vi "HFRR ADV v10.vi"() -> ()   [LabVIEW 2025] (continued)
            n1538 = Add(x=w2006, y=w2020) -> (x+y=w2022:dbl)
            n1539 = call-poly <vilib>:"Mean.vi"("X"=w2043) -> ("mean"=w2044:dbl)  [unwired: 1 out]
            n1540 = Add(x=w1991, y=w1992) -> (x+y=w1990:dbl)
            n1541 = Subtract(x=1.0 ("y"), y=w2032) -> (x-y=w2030:dbl)
            n1542 = local write "TEMP"(w1982) -> ()
            n1543 = Multiply(x=w2030, y=w2029) -> (x*y=w2028:dbl)
            n1544 = Multiply(x=w2022, y=w2032) -> (x*y=w2033:dbl)
            n1545 = Not A Number/Path/Refnum?(number/path/refnum=w1990) -> (NaN/Path/Refnum?=w2000:bool)
            n1546 = Subtract(x=w2043, y=w2044) -> (x-y=w2015:dbl[])
            n1547 = local read "FRICVALZ"() -> (w2053:dbl)
            n1548 = case shown="True" "Camera Button" {
              tunnel: w2010 -> [_ w2072]
              tunnel: "Standard Temp. ( °c )" -> [_ w2071]
              frame False {
              }
              frame True {
                n1549 = Build Array(w2071, w2072) -> (w2070:dbl[])
                n1550 = local write "Camera Button"(FALSE ("Boolean 4")) -> ()
                n1551 = local read "Captured Values"() -> (w2069:dbl[][])
                n1552 = Build Array (concatenate)(w2069, w2070) -> (w2067:dbl[][])
                n1553 = local write "Captured Values"(w2067) -> ()
              }
            }
            n1554 = Compound Arithmetic op=OR("FRICVALZ 4", "FRICVALZ 3", "FRICVALZ 2") -> (w1984:bool)
            n1555 = Add(x=w2033, y=w2028) -> (x+y=w2026:dbl)
            n1556 = Absolute Value(x=w2015) -> (abs(x)=w2048:dbl[])
            n1557 = call-poly <vilib>:"RMS.vi"("X"=w2015) -> ("rms value"=w2014:dbl)  [unwired: 1 out]
            n1558 = Select(t=0.0, s=w2000, f=w1990) -> (s? t:f=w1997:dbl)
            n1559 = call-poly <vilib>:"Mean.vi"("X"=w2048) -> ()  [unwired: 2 out]
            n1560 = local read "FF 2"() -> (w2055:dbl)
            n1561 = case shown="True" w1984 {
              tunnel: w2014 -> [_ w2077]
              frame False {
              }
              frame True {
                w2076 = FALSE ("FRICVALZ")
                n1562 = local write "FRICVALZ 3"(w2076) -> ()
                n1563 = local write "FRICVALZ 2"(w2076) -> ()
                n1564 = local write "FRICVALZ 4"(w2076) -> ()
                "FRICVALZ" <- w2077
              }
            }
            n1565 = Subtract(x=w2014, y=w2053) -> (x-y=w2047:dbl)
            n1566 = Not A Number/Path/Refnum?(number/path/refnum=w2026) -> (NaN/Path/Refnum?=w2027:bool)
            n1567 = In Range and Coerce(upper limit=100.0, x=w1997, lower limit=0.0) -> ()  [unwired: 2 out]
            n1568 = Select(t=0.0, s=w2027, f=w2026) -> (s? t:f=w1987:dbl)
            "AIR TEMP" <- w1987
            n1569 = Multiply(x=w2047, y=0.1 ("FF fil1")) -> (x*y=w2059:dbl)
            n1570 = Multiply(x=0.9 ("FF fil2"), y=w2055) -> (x*y=w2058:dbl)
            n1571 = disable-structure shown="Disabled" {
              frame Disabled {
                n1572 = local read "NORMAL LOAD"() -> ()  [unwired: 1 out]
              }
              frame Enabled {
              }
            }
            n1573 = call "Elapsed Time11"("Time Target (s)"=1.0) -> ("Time has Elapsed"=w1989:bool)  [unwired: 11 in, 7 out]
            n1574 = Add(x=w2059, y=w2058) -> (x+y=w1977:dbl)
            "FF 2" <- w1977
            "FF 4" <- w1977
            n1575 = case shown="True" w1989 {
              tunnel: w1987 -> [_ w2061]
              frame False {
              }
              frame True {
                "AirT" <- w2061
              }
            }
            n1576 = local read "TEMP"() -> (w2052:dbl)
            n1577 = local write "FF 3"(w1977) -> ()
            n1578 = Not A Number/Path/Refnum?(number/path/refnum=w1977) -> (NaN/Path/Refnum?=w2050:bool)
            n1579 = Divide(x=w1977, y=1.96) -> (x/y=w2017:dbl)
            n1580 = Not A Number/Path/Refnum?(number/path/refnum=w2052) -> (NaN/Path/Refnum?=w2051:bool)
            n1581 = Compound Arithmetic op=OR(w2051, w2050) -> (w2049:bool)
            n1582 = Not A Number/Path/Refnum?(number/path/refnum=w2017) -> (NaN/Path/Refnum?=w2018:bool)
            n1583 = case shown="True" w2049 {
              frame False {
              }
              frame True {
                n1584 = local write "TEMP"(0.0 ("TEMP")) -> ()
                n1585 = local write "FF 2"(0.0 ("FF 2")) -> ()
                n1586 = local write "reinit"(TRUE ("reinit")) -> ()
              }
            }
            n1587 = Select(t=0.0, s=w2018, f=w2017) -> (s? t:f=w1978:dbl)
            "COF 2" <- w1978
            n1588 = local write "COF 3"(w1978) -> ()
          }
          frame #4 {
            n1589 = flat-sequence {
              frame #0 {
                n1590 = Wait (ms)(milliseconds to wait=u32 100) -> ()  [unwired: 1 out]
              }
              frame #1 {
                n1591 = local write "Lift"(FALSE ("Lift")) -> ()
              }
            }
            n1592 = case shown="True" "Calculate Button" {
              frame False {
              }
              frame True {
                n1593 = local write "Calculate Button"(FALSE ("Boolean 6")) -> ()
                n1594 = local read "Captured Values"() -> (w2088:dbl[][])
                n1595 = Index Array(array=w2088, index (col) #1=0 ("disabled index (col)"), index (col) #2=1 ("index (col)")) -> (element #1=w2086:dbl[], element #2=w2084:dbl[])  [unwired: 2 in]
                n1596 = call <vilib>:"Linear Fit.vi"("Y"=w2086, "X"=w2084) -> ("Best Linear Fit"=→"Best Fit":dbl[], "slope"=w2080:dbl, "intercept"=w2079:dbl)  [unwired: 9 in, 2 out]
                "Slope" <- w2080
                "Intercept" <- w2079
                n1597 = local read "Calibrating"() -> (w2081:string)
                n1598 = case shown="\"1\"" w2081 {
                  tunnel: w2080 -> [w2090 w2092]
                  tunnel: w2079 -> [w2089 w2091]
                  frame "0", Default {
                    n1599 = local write "TEMPERATURE :"(w2090) -> ()
                    n1600 = local write "TEMP INTERCEPT:"(w2089) -> ()
                  }
                  frame "1" {
                    n1601 = local write "AIR TEMPERATURE :"(w2092) -> ()
                    n1602 = local write "AIR TEMP INTERCEPT:"(w2091) -> ()
                  }
                }
              }
            }
          }
        }
      }
    }
    n1603 = Wait (ms)(milliseconds to wait=u32 50) -> ()  [unwired: 1 out]
    n1604 = local read "Quit"() -> (w1882:bool)
    "Rate" <- 2500.0 ("No of Samples")
    "Humid Last buf" <- dbl[] [0.0, 0.0, 0.0, 0.0] ("Humid Last buf")
  }
  n1605 = while {
    tunnel: w60 -> [_]
    tunnel: [w2122] -> _
    tunnel: [w2097] -> w57
    i -> [w2122]
    stop <- w2097 stop-if-true
    # "C:\\LAB-IQ-NXT\\Scar View.exe"
    n1606 = local read "OK Button 16"() -> (w2111:bool)
    n1607 = local read "Re-Initialise"() -> (w2107:bool)
    n1608 = local read "Main Tab"() -> (w2103:T2)
    n1609 = local read "service 3"() -> (w2104:bool)
    n1610 = local read "OPEN 6"() -> (w2106:bool)
    n1611 = local read "EDIT 2"() -> (w2109:bool)
    n1612 = flat-sequence {
      frame #0 {
        n1613 = local read "SAVE 2"() -> (w2725:bool)
        n1614 = stacked-sequence {
          frame #0 {
            n1615 = local read "EDIT"() -> (w2779:bool)
            n1616 = case shown="True" w2779 {
              tunnel: [u8 2 ("Disabled") u8 0 ("Disabled")] -> _
              frame False {
                w2781 = FALSE
                n1617 = local write "Password"("") -> ()
                n1618 = property on="SrvM CP" class="Bool (strict)"("Visible"=w2781) -> ()  [unwired: 2 in, 2 out]
                n1619 = property on="message" class="Str"("Visible"=w2781) -> ()  [unwired: 2 in, 2 out]
                n1620 = local write "x = y?"(w2781) -> ()
                n1621 = property on="Password" class="Str"("Visible"=w2781) -> ()  [unwired: 2 in, 2 out]
                n1622 = property on="ENTER THE NEW PASSWORD" class="Str"("Visible"=w2781) -> ()  [unwired: 2 in, 2 out]
                n1623 = property on="ENTER CURRENT PASSWORD" class="Str"("Visible"=w2781) -> ()  [unwired: 2 in, 2 out]
                n1624 = local write "SrvM CP"(w2781) -> ()
              }
              frame True {
                w2784 = TRUE
                n1625 = property on="SrvM CP" class="Bool (strict)"("Visible"=w2784) -> ()  [unwired: 2 in, 2 out]
                n1626 = property on="Password" class="Str"("Visible"=w2784) -> ()  [unwired: 2 in, 2 out]
              }
            }
            "dipl pwd" <- "@143$\n" ("dipl pwd")
          }
          frame #1 {
            # "Gain password"
            n1627 = String To Byte Array(string="ENTER CURRENT PASSWORD") -> (unsigned byte array=w2789:u8[])
            n1628 = Search 1D Array(1D array=w2789, element=u8 10) -> (index of element=w2792:i32)  [unwired: 1 in]
            n1629 = Index Array(array=w2789, index=w2792) -> (element=w2788:u8)
            n1630 = Equal?(x=w2788, y=10) -> (x = y?=w2786:bool)
            n1631 = case shown="True" w2786 {
              frame False {
                n1632 = property on="ENTER THE NEW PASSWORD" class="Str"("Visible"=FALSE) -> ()  [unwired: 2 in, 2 out]
              }
              frame True {
                # "password"
                # "change password logic"
                n1633 = local read "ENTER CURRENT PASSWORD"() -> (w2805:string)
                n1634 = local read "dipl pwd"() -> (w2799:string)
                n1635 = String To Byte Array(string=w2805) -> (unsigned byte array=w2807:u8[])
                n1636 = String To Byte Array(string=w2799) -> (unsigned byte array=w2800:u8[])
                n1637 = Array Size(array=w2807) -> (size(s)=w2804:i32)
                n1638 = Array Size(array=w2800) -> (size(s)=w2802:i32)
                n1639 = for {
                  N: w2804 -> [_]
                  tunnel: w2807 -> [w2831]
                  tunnel: [w2829] -> w2808 mode=indexing
                  tunnel: w2804 -> [w2823]
                  i -> [w2824]
                  n1640 = Decrement(x=w2823) -> (x-1=w2821:i32)
                  n1641 = Equal?(x=w2824, y=w2821) -> (x = y?=w2822:bool)
                  n1642 = Index Array(array=w2831, index=w2824) -> (element=w2825:u8)
                  n1643 = Number To Decimal String(number=w2825) -> (decimal integer string=w2830:string)  [unwired: 1 in]
                  n1644 = Select(t="", s=w2822, f="\r") -> (s? t:f=w2827:string)
                  n1645 = Concatenate Strings(w2830, w2827) -> (w2829:string)
                }
                n1646 = for {
                  N: w2802 -> [_]
                  tunnel: w2800 -> [w2819]
                  tunnel: [w2817] -> w2801 mode=indexing
                  tunnel: w2802 -> [w2814]
                  i -> [w2815]
                  n1647 = Decrement(x=w2814) -> (x-1=w2813:i32)
                  n1648 = Equal?(x=w2815, y=w2813) -> (x = y?=w2812:bool)
                  n1649 = Index Array(array=w2819, index=w2815) -> (element=w2818:u8)
                  n1650 = Number To Decimal String(number=w2818) -> (decimal integer string=w2816:string)  [unwired: 1 in]
                  n1651 = Select(t="", s=w2812, f="\r") -> (s? t:f=w2809:string)
                  n1652 = Concatenate Strings(w2816, w2809) -> (w2817:string)
                }
                n1653 = local read "string"() -> (w2806:string)
                n1654 = Concatenate Strings(w2801) -> (w2795:string)
                n1655 = Concatenate Strings(w2806) -> (w2803:string)
                n1656 = Concatenate Strings(w2808) -> (w2796:string)
                n1657 = Equal?(x=w2796, y=w2803) -> (x = y?=w2798:bool)
                n1658 = Equal?(x=w2796, y=w2795) -> (x = y?=w2794:bool)
                n1659 = Or(x=w2798, y=w2794) -> (x .or. y?=w2797:bool)
                n1660 = case shown="True" w2797 {
                  frame False {
                  }
                  frame True {
                    n1661 = property on="ENTER THE NEW PASSWORD" class="Str"("Visible"=TRUE) -> ()  [unwired: 2 in, 2 out]
                  }
                }
              }
            }
          }
          frame #2 {
            n1662 = String To Byte Array(string="ENTER THE NEW PASSWORD") -> (unsigned byte array=w2834:u8[])
            n1663 = Search 1D Array(1D array=w2834, element=u8 10) -> (index of element=w2838:i32)  [unwired: 1 in]
            n1664 = Index Array(array=w2834, index=w2838) -> (element=w2836:u8)
            n1665 = Equal?(x=w2836, y=10) -> (x = y?=w2833:bool)
            n1666 = case shown="False" w2833 {
              frame False {
              }
              frame True {
                n1667 = local write "EDIT"(FALSE) -> ()
                n1668 = local write "SrvM CP"(FALSE) -> ()
                n1669 = local read "ENTER THE NEW PASSWORD"() -> (w2841:string)
                n1670 = String To Byte Array(string=w2841) -> (unsigned byte array=w2846:u8[])
                n1671 = Array Size(array=w2846) -> (size(s)=w2843:i32)
                n1672 = for {
                  N: w2843 -> [_]
                  tunnel: w2846 -> [w2859]
                  tunnel: [w2856] -> w2848 mode=indexing
                  tunnel: w2843 -> [w2851]
                  i -> [w2849]
                  n1673 = Decrement(x=w2851) -> (x-1=w2852:i32)
                  n1674 = Equal?(x=w2849, y=w2852) -> (x = y?=w2853:bool)
                  n1675 = Index Array(array=w2859, index=w2849) -> (element=w2858:u8)
                  n1676 = Number To Decimal String(number=w2858) -> (decimal integer string=w2857:string)  [unwired: 1 in]
                  n1677 = Select(t="", s=w2853, f="\r") -> (s? t:f=w2850:string)
                  n1678 = Concatenate Strings(w2857, w2850) -> (w2856:string)
                }
                n1679 = local read "file path"() -> (w2840:path)
                n1680 = Concatenate Strings(w2848) -> (w2842:string)
                n1681 = Delete(path (use dialog)=w2840) -> (deleted path=w2844:path)  [unwired: 4 in, 2 out]
                n1682 = call <vilib>:"Write Characters To File.vi"("append to file? (new file:F)"=FALSE, "character string"=w2842, "file path (dialog if empty)"=w2844) -> ()  [unwired: 2 in, 1 out]
              }
            }
          }
          frame #3 {
            n1683 = case shown="True" "SrvM CP" {
              frame False {
                w2862 = ""
                n1684 = local write "ENTER CURRENT PASSWORD"(w2862) -> ()
                n1685 = local write "ENTER THE NEW PASSWORD"(w2862) -> ()
                n1686 = property on="ENTER CURRENT PASSWORD" class="Str"("Visible"=FALSE) -> ()  [unwired: 2 in, 2 out]
              }
              frame True {
                n1687 = property on="ENTER THE NEW PASSWORD" class="Str"() -> ("Visible"=w2863:bool)  [unwired: 2 in, 2 out]
                n1688 = Not(x=w2863) -> (.not. x?=w2864:bool)
                n1689 = property on="ENTER CURRENT PASSWORD" class="Str"("Visible"=w2864) -> ()  [unwired: 2 in, 2 out]
              }
            }
          }
          frame #4 {
            n1690 = String To Byte Array(string="Password") -> (unsigned byte array=w2871:u8[])
            n1691 = Search 1D Array(1D array=w2871, element=u8 10) -> (index of element=w2869:i32)  [unwired: 1 in]
            n1692 = Index Array(array=w2871, index=w2869) -> (element=w2870:u8)
            n1693 = Equal?(x=w2870, y=10) -> (x = y?=w2866:bool)
            n1694 = case shown="True" w2866 {
              frame False {
              }
              frame True {
                # "password"
                # "password"
                n1695 = local read "Password"() -> (w2884:string)
                n1696 = String To Byte Array(string=w2884) -> (unsigned byte array=w2887:u8[])
                n1697 = String To Byte Array(string="@143$\n") -> (unsigned byte array=w2873:u8[])
                n1698 = Array Size(array=w2887) -> (size(s)=w2882:i32)
                n1699 = Array Size(array=w2873) -> (size(s)=w2878:i32)
                n1700 = for {
                  N: w2882 -> [_]
                  tunnel: w2887 -> [w2921]
                  tunnel: [w2919] -> w2888 mode=indexing
                  tunnel: w2882 -> [w2916]
                  i -> [w2917]
                  n1701 = Decrement(x=w2916) -> (x-1=w2915:i32)
                  n1702 = Index Array(array=w2921, index=w2917) -> (element=w2920:u8)
                  n1703 = Equal?(x=w2917, y=w2915) -> (x = y?=w2914:bool)
                  n1704 = Number To Decimal String(number=w2920) -> (decimal integer string=w2918:string)  [unwired: 1 in]
                  n1705 = Select(t="", s=w2914, f="\r") -> (s? t:f=w2911:string)
                  n1706 = Concatenate Strings(w2918, w2911) -> (w2919:string)
                }
                n1707 = for {
                  N: w2878 -> [_]
                  tunnel: w2873 -> [w2932]
                  tunnel: [w2930] -> w2876 mode=indexing
                  tunnel: w2878 -> [w2927]
                  i -> [w2928]
                  n1708 = Decrement(x=w2927) -> (x-1=w2926:i32)
                  n1709 = Index Array(array=w2932, index=w2928) -> (element=w2931:u8)
                  n1710 = Equal?(x=w2928, y=w2926) -> (x = y?=w2925:bool)
                  n1711 = Number To Decimal String(number=w2931) -> (decimal integer string=w2929:string)  [unwired: 1 in]
                  n1712 = Select(t="", s=w2925, f="\r") -> (s? t:f=w2922:string)
                  n1713 = Concatenate Strings(w2929, w2922) -> (w2930:string)
                }
                n1714 = local read "file path"() -> (w2872:path)
                n1715 = call <vilib>:"Read Characters From File.vi"("file path (dialog if empty)"=w2872) -> ("character string"=w2886:string)  [unwired: 5 in, 3 out]
                "string" <- w2886
                n1716 = flat-sequence {
                  tunnel: [w2889] -> w2883
                  frame #0 {
                    w2889 = ""
                    n1717 = local write "Password"(w2889) -> ()
                  }
                }
                n1718 = Concatenate Strings(w2876) -> (w2877:string)
                n1719 = Concatenate Strings(w2886) -> (w2885:string)
                n1720 = Concatenate Strings(w2888) -> (w2880:string)
                n1721 = Equal?(x=w2880, y=w2885) -> (x = y?=w2875:bool)
                n1722 = Equal?(x=w2880, y=w2877) -> (x = y?=w2881:bool)
                n1723 = Or(x=w2875, y=w2881) -> (x .or. y?=w2874:bool)
                "x = y?" <- w2874
                n1724 = case shown="True" w2874 {
                  selector: w2874 -> [w2891 _]
                  tunnel: w2883 -> [_ _]
                  frame False {
                    n1725 = And(x=w2891, y=TRUE ("Visible")) -> (x .and. y?=w2892:bool)
                    n1726 = property on="message" class="Str"("Visible"=w2892) -> ()  [unwired: 2 in, 2 out]
                  }
                  frame True {
                    n1727 = control-ref of="This VI"() -> (w2903:refnum<vi>)
                    n1728 = property class="VI"(reference=w2903) -> (reference out=w2894:refnum<vi>, error out=w2898:errorcluster, "Panel"=w2902:refnum<vi>)  [unwired: 1 in]
                    n1729 = property on="message" class="Str"("Visible"=FALSE) -> ()  [unwired: 2 in, 2 out]
                    n1730 = property class="Pnl"(reference=w2902, error in=w2898) -> (reference out=w2896:refnum<vi>, error out=w2899:errorcluster, "Panes[]"=w2901:refnum<vi>[])
                    n1731 = for {
                      tunnel: w2901 -> [w2910] mode=indexing
                      tunnel: T18."Always On" ("Horizontal Scrollbar Visibility") -> [w2909]
                      tunnel: w2899 -> [w2906]
                      tunnel: [w2905] -> w2897
                      n1732 = property class="Pane"(reference=w2910, error in=w2906, "HorizScrollbarVisibility"=w2909) -> (reference out=w2907:refnum<vi>, error out=w2908:errorcluster)
                      n1733 = Close Reference(reference=w2907, error in (no error)=w2908) -> (error out=w2905:errorcluster)
                    }
                    n1734 = Close Reference(reference=w2896, error in (no error)=w2897) -> (error out=w2895:errorcluster)
                    n1735 = Close Reference(reference=w2894, error in (no error)=w2895) -> (error out=→"error out 6":errorcluster)
                  }
                }
              }
            }
          }
        }
        n1736 = local read "x = y?"() -> (w2731:bool)
        n1737 = local read "HUMIDITY: 2"() -> (w2733:dbl)
        n1738 = local read "HUMIDITY:"() -> (w2732:dbl)
        n1739 = property on="Port 2 Error" class="Clust (strict)"("Visible"="EDIT") -> ()  [unwired: 2 in, 2 out]
        n1740 = property on="Port 1 Error" class="Clust (strict)"("Visible"="EDIT") -> ()  [unwired: 2 in, 2 out]
        n1741 = case shown="True" "SrvM CP 2" {
          frame False {
          }
          frame True {
            n1742 = local write "SrvM CP 2"(FALSE ("SrvM CP 2")) -> ()
            n1743 = local read "HUMIDITY: 2"() -> (w2772:dbl)
            n1744 = local read "TEMP INTERCEPT: 2"() -> (w2771:dbl)
            n1745 = local read "DISPLACEMENT : 4"() -> (w2775:dbl)
            n1746 = local read "TEMPERATURE : 2"() -> (w2774:dbl)
            n1747 = local read "STROKE GAIN : 2"() -> (w2776:dbl)
            n1748 = local read "FRIC. FORCE : 2"() -> (w2777:dbl)
            n1749 = local read "AIR TEMP INTERCEPT: 2"() -> (w2770:dbl)
            n1750 = local read "AIR TEMPERATURE : 2"() -> (w2773:dbl)
            n1751 = local write "HUMIDITY:"(w2772) -> ()
            n1752 = local write "AIR TEMP INTERCEPT:"(w2771) -> ()
            n1753 = local write "TEMPERATURE :"(w2774) -> ()
            n1754 = local write "FRIC. FORCE :"(w2777) -> ()
            n1755 = local write "STROKE GAIN :"(w2776) -> ()
            n1756 = local write "DISPLACEMENT :"(w2775) -> ()
            n1757 = local write "AIR TEMPERATURE :"(w2773) -> ()
            n1758 = local write "TEMP INTERCEPT:"(w2770) -> ()
          }
        }
        n1759 = Or(x="SAVE", y=w2725) -> (x .or. y?=w2726:bool)
        n1760 = And(x="EDIT", y=w2731) -> (x .and. y?=w2729:bool)
        n1761 = local read "DISPLACEMENT : 4"() -> (w2742:dbl)
        n1762 = local read "TEMPERATURE : 2"() -> (w2740:dbl)
        n1763 = local read "STROKE GAIN : 2"() -> (w2746:dbl)
        n1764 = local read "DISPLACEMENT :"() -> (w2741:dbl)
        n1765 = local read "FRIC. FORCE : 2"() -> (w2749:dbl)
        n1766 = local read "TEMPERATURE :"() -> (w2738:dbl)
        n1767 = local read "STROKE GAIN :"() -> (w2745:dbl)
        n1768 = local read "FRIC. FORCE :"() -> (w2748:dbl)
        n1769 = case shown="True" w2729 {
          tunnel: [u8 2 ("Disabled") u8 0 ("Disabled")] -> w2728
          tunnel: [w3119 TRUE ("Visible")] -> w2727
          frame False {
            w3119 = FALSE ("Visible")
            n1770 = local write "EDIT 2"(w3119) -> ()
          }
          frame True {
          }
        }
        n1771 = case shown="True" w2726 {
          frame False {
          }
          frame True {
            n1772 = stacked-sequence {
              seq-local: [w2949 _ _] -> [_ w3113 _]
              frame #0 {
                (unwired) i16 5 ("precision (6)")
                # "[CH1]    - FF\n[CH2]   - TEMPERATURE\n[CH3]    - Humidity\n[CH4]    - AIR TEMP\n[CH5]\\- Visa Uno\n[CH6] \\- Visa Due\n[CH7]  \\- file path\n[CH8]   - Displacement Gain\n[CHA]   - Stroke Gain\n[CHB]   - Stroke PID Gain\n[CHC]   -Language Selection\n[CHD]   -Power +\n[CHE]   -Power_\n[CHF]   -Heater\n[CHG]   -Humidity Wet\n[CHH]   -Humidity Dry\n[CHI]   -Integral Time"
                n1773 = local read "Stroke PID Gains"() -> (w3000:T9)
                n1774 = Unbundle By Name(w3000) -> ("Proportional Gain (Kc)"=w2999:dbl, "Integral Time (Ti, min)"=w2941:dbl)
                n1775 = Number To Fractional String(number=w2941, width (-)=i16 10 ("precision (6)"), precision (6)=i16 5) -> (F-format string=w2945:string)  [unwired: 1 in]
                n1776 = local read "Language Selection"() -> (w2997:enum16{"English", "Russian"})
                n1777 = local read "CH-HUMIDITY WET"() -> (w2955:u16)
                n1778 = local read "CH-HUMIDITY DRY"() -> (w2952:u16)
                n1779 = local read "STROKE GAIN :"() -> (w2933:dbl)
                n1780 = local read "CH-POWER +"() -> (w2964:u16)
                n1781 = local read "CH-POWER -"() -> (w2961:u16)
                n1782 = local read "CH-HEATER"() -> (w2958:u16)
                n1783 = local read "AIR TEMPERATURE :"() -> (w2936:dbl)
                n1784 = Concatenate Strings("[CHI]" ("string"), w2945, "-Integral Time " ("string"), "\r") -> (w2942:string)
                n1785 = local read "DISPLACEMENT :"() -> (w2934:dbl)
                n1786 = local read "TEMPERATURE :"() -> (w2937:dbl)
                n1787 = local read "FRIC. FORCE :"() -> (w2938:dbl)
                n1788 = local read "HUMIDITY:"() -> (w2935:dbl)
                n1789 = Path To String(path="File Path") -> (string=w3022:string)
                n1790 = Number To Fractional String(number=w2933, width (-)=i16 10 ("precision (6)"), precision (6)=i16 5) -> (F-format string=w3013:string)  [unwired: 1 in]
                n1791 = Number To Fractional String(number=w2999, width (-)=i16 10 ("precision (6)"), precision (6)=i16 5) -> (F-format string=w3001:string)  [unwired: 1 in]
                n1792 = Number To Fractional String(number=w2997, width (-)=i16 10 ("precision (6)"), precision (6)=i16 5) -> (F-format string=w2993:string)  [unwired: 1 in]
                n1793 = Number To Fractional String(number=w2964, width (-)=i16 10 ("precision (6)"), precision (6)=i16 5) -> (F-format string=w2987:string)  [unwired: 1 in]
                n1794 = Number To Fractional String(number=w2961, width (-)=i16 10 ("precision (6)"), precision (6)=i16 5) -> (F-format string=w2984:string)  [unwired: 1 in]
                n1795 = Number To Fractional String(number=w2958, width (-)=i16 10 ("precision (6)"), precision (6)=i16 5) -> (F-format string=w2979:string)  [unwired: 1 in]
                n1796 = Number To Fractional String(number=w2955, width (-)=i16 10 ("precision (6)"), precision (6)=i16 5) -> (F-format string=w2976:string)  [unwired: 1 in]
                n1797 = Number To Fractional String(number=w2952, width (-)=i16 10 ("precision (6)"), precision (6)=i16 5) -> (F-format string=w2971:string)  [unwired: 1 in]
                n1798 = local read "Com Port 1"() -> (w2940:refnum<visa-resource-name>)
                n1799 = local read "Com Port 2"() -> (w2939:refnum<visa-resource-name>)
                n1800 = Concatenate Strings(w3022, "\\" ("string")) -> (w3021:string)
                n1801 = Number To Fractional String(number=w2938, width (-)=i16 10 ("precision (6)"), precision (6)=i16 5) -> (F-format string=w3054:string)  [unwired: 1 in]
                n1802 = Number To Fractional String(number=w2937, width (-)=i16 10 ("precision (6)"), precision (6)=i16 5) -> (F-format string=w3053:string)  [unwired: 1 in]
                n1803 = Number To Fractional String(number=w2935, width (-)=i16 10 ("precision (6)"), precision (6)=i16 5) -> (F-format string=w3047:string)  [unwired: 1 in]
                n1804 = Number To Fractional String(number=w2936, width (-)=i16 10 ("precision (6)"), precision (6)=i16 5) -> (F-format string=w3041:string)  [unwired: 1 in]
                n1805 = Number To Fractional String(number=w2934, width (-)=i16 10 ("precision (6)"), precision (6)=i16 5) -> (F-format string=w3014:string)  [unwired: 1 in]
                n1806 = Concatenate Strings("[CHA]" ("string"), w3013, "- Stroke Gain" ("string"), "\r") -> (w3007:string)
                n1807 = Concatenate Strings("[CHB]" ("string"), w3001, "- Stroke PID Gain" ("string"), "\r") -> (w2998:string)
                n1808 = Concatenate Strings("[CHC]" ("string"), w2993, "-Language Selection" ("string"), "\r") -> (w2990:string)
                n1809 = Concatenate Strings("[CHD]" ("string"), w2987, "-Power +" ("string"), "\r") -> (w2969:string)
                n1810 = Concatenate Strings("[CHG]" ("string"), w2976, "-Humidity Wet" ("string"), "\r") -> (w2966:string)
                n1811 = Concatenate Strings("[CHH]" ("string"), w2971, "-Humidity Dry" ("string"), "\r") -> (w2965:string)
                n1812 = Concatenate Strings("[CH1]" ("string"), w3054, " - FF" ("string"), "\r") -> (w3052:string)
                n1813 = Concatenate Strings("[CH2]" ("string"), w3053, " - TEMPERATURE" ("string"), "\r") -> (w3051:string)
                n1814 = Concatenate Strings("[CH3]" ("string"), w3047, " - Humidity" ("string"), "\r") -> (w3044:string)
                n1815 = Concatenate Strings("[CH4]" ("string"), w3041, " - AIR TEMP" ("string"), "\r") -> (w3037:string)
                n1816 = Concatenate Strings("[CH5]" ("string"), w2940, "- Visa Uno" ("string"), "\r") -> (w3030:string)
                n1817 = Concatenate Strings("[CH6]" ("string"), w2939, "- Visa Due" ("string"), "\r") -> (w3025:string)
                n1818 = Concatenate Strings("[CH7]" ("string"), w3021, "- file path" ("string"), "\r") -> (w3024:string)
                n1819 = Concatenate Strings("[CH8]" ("string"), w3014, "- Displacement Gain" ("string"), "\r") -> (w3017:string)
                n1820 = Concatenate Strings("[CHE]" ("string"), w2984, "-Power_" ("string"), "\r") -> (w2968:string)
                n1821 = Concatenate Strings("[CHF]" ("string"), w2979, "-Heater" ("string"), "\r") -> (w2967:string)
                n1822 = Concatenate Strings(w3052, w3051, w3044, w3037, w3030, w3025, w3024, w3017, w3007, w2998, w2990, w2969, w2968, w2967, w2966, w2965, w2942) -> (w2949:string)
                "gain" <- w2949
              }
              frame #1 {
                n1823 = local read "Camera Port :"() -> (w3066:string)
                n1824 = local read "TEMP INTERCEPT:"() -> (w3075:dbl)
                n1825 = local read "AIR TEMP INTERCEPT:"() -> (w3076:dbl)
                n1826 = local read "C3 :"() -> (w3074:refnum<visa-resource-name>)
                n1827 = local read "LvdtOff"() -> (w3078:dbl)
                n1828 = Number To Fractional String(number=w3075, width (-)=i16 10 ("precision (6)"), precision (6)=i16 5) -> (F-format string=w3101:string)  [unwired: 1 in]
                n1829 = local read "Com Port 3"() -> (w3085:refnum<visa-resource-name>)
                n1830 = Concatenate Strings("[CH8]" ("string"), w3066, "- Visa Camera" ("string"), "\r") -> (w3065:string)
                n1831 = Concatenate Strings("[CH7]" ("string"), w3074, "- Visa Humidity" ("string"), "\r") -> (w3070:string)
                n1832 = Number To Fractional String(number=w3076, width (-)=i16 10 ("precision (6)"), precision (6)=i16 5) -> (F-format string=w3108:string)  [unwired: 1 in]
                n1833 = Number To Fractional String(number=w3078, width (-)=i16 10 ("precision (6)"), precision (6)=i16 5) -> (F-format string=w3082:string)  [unwired: 1 in]
                n1834 = Concatenate Strings("[CHK]" ("string"), w3101, "-TEMP INTERCEPT" ("string"), "\r") -> (w3097:string)
                n1835 = Concatenate Strings("[SNO]" ("string"), "S.NO", "-" ("string"), "\r") -> (w3093:string)
                n1836 = Concatenate Strings("[CHI]" ("string"), w3082, "-LVDT Position Offset" ("string"), "\r") -> (w3077:string)
                n1837 = Concatenate Strings("[CHJ]" ("string"), w3108, "-AIR TEMP INTERCEPT" ("string"), "\r") -> (w3098:string)
                n1838 = Concatenate Strings("[CHL]" ("string"), w3085, "- Visa humid" ("string"), "\r") -> (w3088:string)
                n1839 = String To Path(string="C:\\LAB-IQ\\calibrate WO 2465.dcf") -> (path=w3086:path)
                n1840 = Concatenate Strings(w3113, w3098, w3097, w3093, w3088, w3077, w3070, w3065) -> (w3112:string)
                n1841 = call <vilib>:"Write Characters To File.vi"("append to file? (new file:F)"=FALSE, "character string"=w3112, "file path (dialog if empty)"=w3086) -> ()  [unwired: 2 in, 1 out]
              }
              frame #2 {
                n1842 = local write "Lan flag"(0.0 ("Lan flag")) -> ()
                n1843 = local write "conststatus"(0.0 ("rpm value : 2")) -> ()
                n1844 = local write "SAVE"(FALSE ("OK Button 14")) -> ()
                n1845 = local write "Re-Initialise"(TRUE ("Re-Initialise")) -> ()
                n1846 = local write "SAVE 2"(FALSE ("SAVE 2")) -> ()
              }
            }
          }
        }
        n1847 = Subtract(x=w2733, y=w2732) -> (x-y=w2734:dbl)
        n1848 = local read "AIR TEMPERATURE : 2"() -> (w2737:dbl)
        n1849 = local read "AIR TEMPERATURE :"() -> (w2736:dbl)
        n1850 = Divide(x=w2734, y=w2732) -> (x/y=w2756:dbl)
        n1851 = Subtract(x=w2749, y=w2748) -> (x-y=w2747:dbl)
        n1852 = Subtract(x=w2740, y=w2738) -> (x-y=w2739:dbl)
        n1853 = Subtract(x=w2746, y=w2745) -> (x-y=w2744:dbl)
        n1854 = Subtract(x=w2742, y=w2741) -> (x-y=w2743:dbl)
        n1855 = Subtract(x=w2737, y=w2736) -> (x-y=w2735:dbl)
        n1856 = Divide(x=w2747, y=w2748) -> (x/y=w2767:dbl)
        n1857 = Divide(x=w2739, y=w2738) -> (x/y=w2760:dbl)
        n1858 = Divide(x=w2744, y=w2745) -> (x/y=w2764:dbl)
        n1859 = Divide(x=w2743, y=w2741) -> (x/y=w2763:dbl)
        n1860 = Multiply(x=w2756, y=100.0) -> (x*y=→"HUMIDITY  Calibration Error":dbl)
        n1861 = Divide(x=w2735, y=w2736) -> (x/y=w2759:dbl)
        n1862 = Multiply(x=w2767, y=100.0) -> (x*y=→"FRIC. FORCE Calibration Error":dbl)
        n1863 = Multiply(x=w2760, y=100.0) -> (x*y=→"TEMPERATURE  Calibration Error":dbl)
        n1864 = Multiply(x=w2764, y=100.0) -> (x*y=→"STROKE Calibration Error":dbl)
        n1865 = Multiply(x=w2763, y=100.0) -> (x*y=→"DISPLACEMENT  Calibration Error":dbl)
        n1866 = property on="EDIT 2" class="Bool (strict)"("Visible"=w2727) -> ()  [unwired: 2 in, 2 out]
        n1867 = property on="SAVE" class="Bool (strict)"("Visible"=w2727) -> ()  [unwired: 2 in, 2 out]
        n1868 = property on="SrvM CP" class="Bool (strict)"("Disabled"=w2728) -> ()  [unwired: 2 in, 2 out]
        n1869 = property on="visa due" class="CmbBox"("Disabled"=w2728) -> ()  [unwired: 2 in, 2 out]
        n1870 = property on="LvdtOff" class="DigNum (strict)"("Disabled"=w2728) -> ()  [unwired: 2 in, 2 out]
        n1871 = property on="File Path" class="Path"("Disabled"=w2728) -> ()  [unwired: 2 in, 2 out]
        n1872 = Multiply(x=w2759, y=100.0) -> (x*y=→"AIR TEMPERATURE  Calibration Error":dbl)
        n1873 = property on="Tab Control" class="TabCtl (strict)"("Visible"=w2727) -> ()  [unwired: 2 in, 2 out]
        n1874 = property on="Language Selection" class="Enum (strict)"("Visible"=w2727) -> ()  [unwired: 2 in, 2 out]
        n1875 = property on="Tab Control 7" class="TabCtl (strict)"("Disabled"=w2728) -> ()  [unwired: 2 in, 2 out]
        n1876 = property on="AIR TEMP INTERCEPT:" class="DigNum (strict)"("Disabled"=w2728) -> ()  [unwired: 2 in, 2 out]
        n1877 = property on="CH-POWER -" class="DigNum (strict)"("Disabled"=w2728) -> ()  [unwired: 2 in, 2 out]
        n1878 = property on="CH-POWER +" class="DigNum (strict)"("Disabled"=w2728) -> ()  [unwired: 2 in, 2 out]
        n1879 = property on="AIR TEMPERATURE :" class="DigNum (strict)"("Disabled"=w2728) -> ()  [unwired: 2 in, 2 out]
        n1880 = property on="STROKE GAIN :" class="DigNum (strict)"("Disabled"=w2728) -> ()  [unwired: 2 in, 2 out]
        n1881 = property on="SPEED OUT:" class="DigNum (strict)"("Disabled"=w2728) -> ()  [unwired: 2 in, 2 out]
        n1882 = property on="CH-HUMIDITY DRY" class="DigNum (strict)"("Disabled"=w2728) -> ()  [unwired: 2 in, 2 out]
        n1883 = property on="HUMIDITY:" class="DigNum (strict)"("Disabled"=w2728) -> ()  [unwired: 2 in, 2 out]
        n1884 = property on="CH-HUMIDITY WET" class="DigNum (strict)"("Disabled"=w2728) -> ()  [unwired: 2 in, 2 out]
        n1885 = property on="Stroke PID Gains" class="Clust (strict)"("Disabled"=w2728) -> ()  [unwired: 2 in, 2 out]
        n1886 = property on="TEMPERATURE :" class="DigNum (strict)"("Disabled"=w2728) -> ()  [unwired: 2 in, 2 out]
        n1887 = property on="DISPLACEMENT :" class="DigNum (strict)"("Disabled"=w2728) -> ()  [unwired: 2 in, 2 out]
        n1888 = property on="CH-HEATER" class="DigNum (strict)"("Disabled"=w2728) -> ()  [unwired: 2 in, 2 out]
        n1889 = property on="TEMP INTERCEPT:" class="DigNum (strict)"("Disabled"=w2728) -> ()  [unwired: 2 in, 2 out]
        n1890 = property on="FRIC. FORCE :" class="DigNum (strict)"("Disabled"=w2728) -> ()  [unwired: 2 in, 2 out]
      }
    }
    n1891 = local read "RUN"() -> (w2121:bool)
    n1892 = local read "RUN"() -> (w2119:bool)
    n1893 = disable-structure shown="Disabled" {
      disable-tunnel: [w2136 _] -> w2101
      disable-tunnel: [w2135 _] -> w2099
      frame Disabled {
        n1894 = local read "Temperature before test"() -> (w2129:dbl)
        n1895 = local read "Temperature after test"() -> (w2142:dbl)
        n1896 = case shown="True" "Save Results" {
          frame False {
          }
          frame True {
            w2158 = "\r"
            n1897 = local write "Save Results"(FALSE ("OK Button 5")) -> ()
            n1898 = local read "Temperature before test"() -> (w2196:dbl)
            n1899 = local read "Temperature after test"() -> (w2198:dbl)
            n1900 = local read "Humidity before test"() -> (w2195:dbl)
            n1901 = local read "Humidity after test"() -> (w2197:dbl)
            n1902 = local read "WS1.4"() -> (w2202:dbl)
            n1903 = local read "AVP"() -> (w2200:dbl)
            n1904 = Number To Fractional String(number=w2202, width (-)=i16 6, precision (6)=i16 1) -> (F-format string=w2162:string)  [unwired: 1 in]
            n1905 = local read "MWSD"() -> (w2199:dbl)
            n1906 = local read "String"() -> (w2191:string)
            n1907 = local read "FILE"() -> (w2194:string)
            n1908 = local read "HCF"() -> (w2201:dbl)
            n1909 = Number To Fractional String(number=w2195, width (-)=i16 6, precision (6)=i16 1) -> (F-format string=w2187:string)  [unwired: 1 in]
            n1910 = Number To Fractional String(number=w2196, width (-)=i16 6, precision (6)=i16 1) -> (F-format string=w2184:string)  [unwired: 1 in]
            n1911 = Number To Fractional String(number=w2197, width (-)=i16 6, precision (6)=i16 1) -> (F-format string=w2180:string)  [unwired: 1 in]
            n1912 = Number To Fractional String(number=w2198, width (-)=i16 6, precision (6)=i16 1) -> (F-format string=w2176:string)  [unwired: 1 in]
            n1913 = Number To Fractional String(number=w2200, width (-)=i16 6, precision (6)=i16 3) -> (F-format string=w2169:string)  [unwired: 1 in]
            n1914 = Concatenate Strings(w2191, w2194) -> (w2213:string)
            n1915 = Number To Fractional String(number=w2199, width (-)=i16 6, precision (6)=i16 1) -> (F-format string=w2173:string)  [unwired: 1 in]
            n1916 = Number To Fractional String(number=w2201, width (-)=i16 6, precision (6)=i16 2) -> (F-format string=w2167:string)  [unwired: 1 in]
            n1917 = Concatenate Strings("(" ("string"), w2162, ")Microns" ("string")) -> (w2161:string)
            n1918 = local read "REMARKS"() -> (w2193:string)
            "REMARKS 2" <- w2193
            n1919 = Concatenate Strings("(" ("string"), w2187, " ) % RH," ("string")) -> (w2188:string)
            n1920 = Concatenate Strings(w2167, ")" ("string")) -> (w2165:string)
            n1921 = Concatenate Strings("(" ("string"), w2184, ")  Deg C ," ("string")) -> (w2183:string)
            n1922 = Concatenate Strings("(" ("string"), w2180, " ) % RH," ("string")) -> (w2179:string)
            n1923 = Concatenate Strings("(" ("string"), w2176, ")  Deg C ," ("string")) -> (w2175:string)
            n1924 = Concatenate Strings("(" ("string"), w2173, ")  Microns," ("string")) -> (w2172:string)
            n1925 = Concatenate Strings("(" ("string"), w2169, ")  kPa," ("string")) -> (w2159:string)
            n1926 = Concatenate Strings(w2213, ".dwm" ("Substring")) -> (w2211:string)
            n1927 = String To Path(string=w2211) -> (path=w2210:path)
            n1928 = Concatenate Strings(w2193, w2158, " Humidity before test= " ("Substring"), w2188, w2158, " Temperature before test = " ("Substring"), w2183, w2158, " Humidity after test= " ("Substring"), w2179, w2158, "Temperature after test = " ("Substring"), w2175, w2158, "MSD = " ("Substring"), w2172, w2158, "  AVP = " ("Substring"), w2159, w2158, "  HCF                     =( " ("Substring"), w2165, w2158, " WS1.4                  = " ("Substring"), w2161, w2158) -> (w2157:string)
            "data" <- w2157
            n1929 = call <vilib>:"Write Characters To File.vi"("append to file? (new file:F)"=FALSE, "character string"=w2157, "file path (dialog if empty)"=w2210) -> ()  [unwired: 2 in, 1 out]
            n1930 = Match Pattern(string=w2157, regular expression="!") -> (after substring=→"export":string)  [unwired: 1 in, 3 out]
          }
        }
        n1931 = Add(x=231.864, y=w2129) -> (x+y=w2126:dbl)
        n1932 = Add(x=231.864, y=w2142) -> (x+y=w2139:dbl)
        n1933 = Divide(x=1705.984, y=w2126) -> (x/y=w2127:dbl)
        n1934 = Divide(x=1705.984, y=w2139) -> (x/y=w2140:dbl)
        n1935 = local read "Humidity before test"() -> (w2131:dbl)
        n1936 = local read "Humidity after test"() -> (w2144:dbl)
        n1937 = Subtract(x=8.017352 ("y"), y=w2127) -> (x-y=w2153:dbl)
        n1938 = Subtract(x=8.017352 ("y"), y=w2140) -> (x-y=w2147:dbl)
        n1939 = expression code="10**y"(w2153) -> (w2133:dbl)
        n1940 = expression code="10**y"(w2147) -> (w2146:dbl)
        n1941 = Multiply(x=w2131, y=w2133) -> (x*y=w2132:dbl)
        n1942 = Multiply(x=w2144, y=w2146) -> (x*y=w2145:dbl)
        n1943 = Divide(x=w2132, y=750.0) -> (x/y=w2148:dbl)
        n1944 = Divide(x=w2145, y=750.0) -> (x/y=w2149:dbl)
        n1945 = Add(x=w2148, y=w2149) -> (x+y=w2150:dbl)
        n1946 = Divide(x=w2150, y=2.0) -> (x/y=w2152:dbl)
        n1947 = local write "AVP"(w2152) -> ()
        n1948 = Subtract(x=1.4, y=w2152) -> (x-y=w2135:dbl)
        n1949 = local read "HCF"() -> (w2136:dbl)
      }
      frame Enabled {
      }
    }
    n1950 = case shown="True" "EDIT 3" {
      frame False {
      }
      frame True {
        n1951 = local write "EDIT 3"(FALSE ("EDIT 3")) -> ()
        n1952 = local write "Main Tab"(T2."About" ("Main Tab")) -> ()
      }
    }
    n1953 = case shown="True" w2107 {
      frame False {
      }
      frame True {
        n1954 = local write "Re-Initialise"(FALSE ("Re-Initialise")) -> ()
      }
    }
    n1955 = case shown="False" w2121 {
      frame False {
        n1956 = local read "stopT"() -> (w3126:bool)
        n1957 = case shown="True" w3126 {
          frame False {
          }
          frame True {
            w3127 = FALSE
            n1958 = local write "stopT"(w3127) -> ()
            n1959 = local write "st enable"(w3127) -> ()
          }
        }
      }
      frame True {
        "stopT" <- TRUE
      }
    }
    n1960 = case shown="True" w2119 {
      frame False {
      }
      frame True {
      }
    }
    n1961 = case shown="True" w2109 {
      frame False {
        n1962 = property on="Password 2" class="Str"("Visible"=FALSE) -> ()  [unwired: 2 in, 2 out]
        n1963 = local write "Password 2"("" ("Password")) -> ()
      }
      frame True {
        n1964 = property on="Password 2" class="Str"("Visible"=TRUE) -> ()  [unwired: 2 in, 2 out]
        n1965 = Equal?(x="Password 2", y="HFRR1234") -> (x = y?=w2242:bool)
        n1966 = case shown="True" w2242 {
          tunnel: "Password 2" -> [w2245 _]
          frame False {
            n1967 = String Length(string=w2245) -> (length=w2246:i32)
            n1968 = Greater Than 0?(x=w2246) -> (x > 0?=w2244:bool)
            n1969 = case shown="False" w2244 {
              frame False {
                n1970 = property on="Password 2" class="Str"("Caption.Text"="Password (Advance Setting)") -> ()  [unwired: 2 in, 2 out]
              }
              frame True {
                n1971 = property on="Password 2" class="Str"("Caption.Text"="Incorrect Password!") -> ()  [unwired: 2 in, 2 out]
              }
            }
          }
          frame True {
            n1972 = local write "EDIT 2"(FALSE ("EDIT 2")) -> ()
            n1973 = local write "Password 2"("" ("Password")) -> ()
            n1974 = local write "Main Tab"(T2."Advance" ("Main Tab")) -> ()
            n1975 = local write "Main Dashboard Buttons"(T1."Advance" ("Main Dashboard Buttons")) -> ()
          }
        }
      }
    }
    n1976 = case shown="True" "Prog Uno" {
      frame False {
      }
      frame True {
        n1977 = stacked-sequence {
          frame #0 {
            n1978 = Delete(path (use dialog)=path "C:/LAB-IQ-NXT/UNOCOMPILE.bat" ("working directory")) -> ()  [unwired: 4 in, 3 out]
          }
          frame #1 {
            n1979 = local read "Com Port 1"() -> (w2707:refnum<visa-resource-name>)
            n1980 = Concatenate Strings("cmd.exe /c \"mode " ("command line"), w2707, ":1200,n,8,1\"\n" ("command line")) -> (w2712:string)
            n1981 = Concatenate Strings(w2712, "CD\\\nCD WinDucom\navrdude -C avrdude.conf -v -patmega328p -carduino -P" ("command line"), w2707, " -b115200 -D -Uflash:w:UNO_V20.hex:i\n" ("command line"), "\r") -> (w2714:string)
            "STR" <- w2714
            n1982 = call <vilib>:"Write Characters To File.vi"("append to file? (new file:F)"=FALSE, "character string"=w2714, "file path (dialog if empty)"=path "C:/LAB-IQ/UNOCOMPILE.bat" ("working directory")) -> ()  [unwired: 2 in, 1 out]
          }
          frame #2 {
            n1983 = disable-structure shown="Disabled" {
              frame Disabled {
                w2718 = "cmd.exe  /c \"C:\\LAB-IQ-NXT\\UNOCOMPILE.bat\"" ("string")
                n1984 = local write "Prog Uno"(FALSE ("run minimized? (F)")) -> ()
                n1985 = call <vilib>:"System Exec.vi"("expected output size  (4096)"=u32 65535, "run minimized? (F)"=FALSE, "wait until completion? (T)"=TRUE ("run minimized? (F)"), "working directory"=path "C:/LAB-IQ-NXT", "standard input"=w2718, "command line"=w2718) -> ("error out"=w2717:errorcluster, "standard output"=→"String 42":string)  [unwired: 2 in, 2 out]
                "error out 3" <- w2717
                n1986 = flat-sequence {
                  tunnel: w2717 -> [_]
                  frame #0 {
                  }
                }
              }
              frame Enabled {
              }
            }
          }
        }
      }
    }
    n1987 = case shown="\"CEC F-096-A-06\"" "TEST STANDARD" {
      tunnel: [2.0 ("Set Temp") 0.0 ("Set Temp") 2.0 ("Set Temp") 0.0 ("Set Temp")] -> w2110
      frame "ASTM D6079", Default {
        w2664 = 50.0 ("Hz")
        w2665 = 53.0 ("Set Rh")
        w2667 = 1.0 ("Set Strk")
        w2666 = 60.0 ("Set Temp")
        # "astm hide"
        n1988 = local write "NORMAL LOAD"(200.0 ("NORMAL LOAD")) -> ()
        n1989 = local write "Set Strk"(w2667) -> ()
        n1990 = local write "Set Hz"(w2664) -> ()
        n1991 = local write "Set Temp"(w2666) -> ()
        n1992 = local write "Set Rh"(w2665) -> ()
        n1993 = local write "test time"(75.0 ("test time")) -> ()
        n1994 = local write "Set Stroke:"(w2667) -> ()
        n1995 = local write "Set Humidity:"(w2665) -> ()
        n1996 = local write "Set Frequency:"(w2664) -> ()
        n1997 = local write "Set Temperature:"(w2666) -> ()
        "Test Standard" <- "ASTM D6079" ("Test Standard 2")
      }
      frame "ISO 12156" {
        n1998 = local write "Set Strk"(1.0 ("Set Strk")) -> ()
        n1999 = local write "NORMAL LOAD"(200.0 ("NORMAL LOAD")) -> ()
        n2000 = local write "Set Temp"(60.0 ("Set Temp")) -> ()
        n2001 = local write "test time"(75.0 ("test time")) -> ()
        n2002 = local write "Set Hz"(50.0 ("Hz")) -> ()
        n2003 = local write "Set Rh"(53.0 ("Set Rh")) -> ()
      }
      frame "CEC F-096-A-06" {
        n2004 = local write "Set Strk"(1.0 ("Set Strk")) -> ()
        n2005 = local write "NORMAL LOAD"(200.0 ("NORMAL LOAD")) -> ()
        n2006 = local write "Set Temp"(60.0 ("Set Temp")) -> ()
        n2007 = local write "test time"(75.0 ("test time")) -> ()
        n2008 = local write "Set Hz"(50.0 ("Hz")) -> ()
        n2009 = local write "Set Rh"(53.0 ("Set Rh")) -> ()
      }
      frame "Custom" {
      }
    }
    n2010 = case shown="True" "Prog Due" {
      frame False {
      }
      frame True {
        n2011 = stacked-sequence {
          frame #0 {
            n2012 = Delete(path (use dialog)=path "C:/LAB-IQ/DUECOMPILE.bat" ("working directory")) -> ()  [unwired: 4 in, 3 out]
          }
          frame #1 {
            n2013 = disable-structure shown="Disabled" {
              frame Disabled {
                n2014 = local read "visa due"() -> (w2689:string)
                n2015 = Concatenate Strings("cmd.exe /c \"mode " ("command line"), w2689, ":1200,n,8,1\"\n" ("command line")) -> (w2694:string)
                n2016 = Concatenate Strings(w2694, "CD\\\nCD WinDucom\nTIMEOUT 1\n bossac.exe -i -d --port=" ("command line"), w2689, " -U false -e -w -v -b DUE.bin -R\n" ("command line"), "\r") -> (w2696:string)
                "concatenated string 2" <- w2696
                n2017 = call <vilib>:"Write Characters To File.vi"("append to file? (new file:F)"=FALSE, "character string"=w2696, "file path (dialog if empty)"=path "C:/LAB-IQ-NXT/DUECOMPILE.bat" ("working directory")) -> ()  [unwired: 2 in, 1 out]
              }
              frame Enabled {
              }
            }
          }
          frame #2 {
            # "C:\\LAB-IQ-NXT\\DUECOMPILE.bat"
            n2018 = disable-structure shown="Disabled" {
              frame Disabled {
                w2701 = "cmd.exe  /c \"C:\\LAB-IQ-NXT\\DUECOMPILE.bat\"" ("string")
                n2019 = call <vilib>:"System Exec.vi"("expected output size  (4096)"=u32 65535, "run minimized? (F)"=FALSE, "wait until completion? (T)"=TRUE ("run minimized? (F)"), "working directory"=path "C:/LAB-IQ-NXT", "standard input"=w2701, "command line"=w2701) -> ("error out"=w2700:errorcluster, "standard output"=→"String 44":string)  [unwired: 2 in, 2 out]
                "error out 4" <- w2700
                n2020 = flat-sequence {
                  tunnel: w2700 -> [_]
                  frame #0 {
                  }
                }
              }
              frame Enabled {
              }
            }
            n2021 = local write "Prog Due"(FALSE ("Prog Due")) -> ()
          }
        }
      }
    }
    n2022 = Or(x=w2106, y=w2104) -> (x .or. y?=w2105:bool)
    n2023 = case shown="\"About\"" w2103 {
      tunnel: [T23."Acquire" ("Main Tab") T23."Compare Files" ("Main Tab") T23."About" ("Main Tab")] -> w2117
      frame "Acquire", Default {
      }
      frame "Compare Files" {
      }
      frame "About" {
      }
    }
    n2024 = Or(x=w2111, y="OPEN") -> (x .or. y?=w2112:bool)
    n2025 = case shown="True" w2112 {
      tunnel: w2111 -> [_ w2253]
      frame False {
      }
      frame True {
        n2026 = stacked-sequence {
          tunnel: w2253 -> [_ w2320 _ _]
          frame #0 {
            w2269 = "  " ("String 6")
            n2027 = local write "OPEN"(FALSE ("open")) -> ()
            n2028 = local read "string1 2"() -> (w2257:string)
            n2029 = local read "string1 3"() -> (w2256:string)
            n2030 = local read "string1 4"() -> (w2255:string)
            n2031 = property on="OPEN" class="Bool (strict)"("Visible"=FALSE) -> ()  [unwired: 2 in, 2 out]
            n2032 = local write "String 6"(w2269) -> ()
            n2033 = local write "String 7"(w2269) -> ()
            n2034 = local write "String 8"(w2269) -> ()
            n2035 = local write "String 12"(w2269) -> ()
            n2036 = local read "OK Button 16"() -> (w2254:bool)
            n2037 = String To Path(string=w2257) -> (path=w2265:path)
            n2038 = String To Path(string=w2256) -> (path=w2264:path)
            n2039 = String To Path(string=w2255) -> (path=w2263:path)
            n2040 = case shown="True" w2254 {
              tunnel: [w2270 w2271] -> w2258
              frame False {
                n2041 = local read "string1"() -> (w2270:string)
              }
              frame True {
                n2042 = local read "String Indicator 4"() -> (w2271:string)
              }
            }
            n2043 = Open/Create/Replace File "Open File"(file path (use dialog)=w2265) -> (refnum out=w2261:refnum<file>)  [unwired: 5 in, 2 out]
            n2044 = Open/Create/Replace File "Open File"(file path (use dialog)=w2264) -> (refnum out=w2260:refnum<file>)  [unwired: 5 in, 2 out]
            n2045 = Open/Create/Replace File "Open File"(file path (use dialog)=w2263) -> (refnum out=w2259:refnum<file>)  [unwired: 5 in, 2 out]
            n2046 = while {
              tunnel: w2261 -> [w2283]
              i -> [w2279]
              stop <- w2278 continue-if-true
              (unwired) TRUE ("line mode (F)")
              n2047 = Read from Text File "Read File"(file (use dialog)=w2283) -> (text=w2280:string)  [unwired: 3 in, 3 out]
              n2048 = local write "Numeric 11"(w2279) -> ()
              n2049 = String Length(string=w2280) -> (length=w2282:i32)
              n2050 = Greater?(x=w2282, y=1) -> (0:w2278:bool)
            }
            n2051 = while {
              tunnel: w2260 -> [w2289]
              i -> [w2285]
              stop <- w2284 continue-if-true
              (unwired) TRUE ("line mode (F)")
              n2052 = Read from Text File "Read File"(file (use dialog)=w2289) -> (text=w2286:string)  [unwired: 3 in, 3 out]
              n2053 = local write "Numeric 12"(w2285) -> ()
              n2054 = String Length(string=w2286) -> (length=w2288:i32)
              n2055 = Greater?(x=w2288, y=1) -> (0:w2284:bool)
            }
            n2056 = while {
              tunnel: w2259 -> [w2295]
              i -> [w2291]
              stop <- w2290 continue-if-true
              (unwired) TRUE ("line mode (F)")
              n2057 = Read from Text File "Read File"(file (use dialog)=w2295) -> (text=w2292:string)  [unwired: 3 in, 3 out]
              n2058 = local write "Numeric 13"(w2291) -> ()
              n2059 = String Length(string=w2292) -> (length=w2294:i32)
              n2060 = Greater?(x=w2294, y=1) -> (0:w2290:bool)
            }
            n2061 = String To Path(string=w2258) -> (path=w2266:path)
            n2062 = Open/Create/Replace File "Open File"(file path (use dialog)=w2266) -> (refnum out=w2262:refnum<file>)  [unwired: 5 in, 2 out]
            n2063 = while {
              tunnel: w2262 -> [w2277]
              i -> [w2273]
              stop <- w2272 continue-if-true
              (unwired) TRUE ("line mode (F)")
              n2064 = Read from Text File "Read File"(file (use dialog)=w2277) -> (text=w2274:string)  [unwired: 3 in, 3 out]
              n2065 = local write "Numeric 8"(w2273) -> ()
              n2066 = String Length(string=w2274) -> (length=w2276:i32)
              n2067 = Greater?(x=w2276, y=1) -> (0:w2272:bool)
            }
          }
          frame #1 {
            w2447 = FALSE ("ACTUAL   MERGE")
            # "Sample Temp"
            # "ECR"
            # "COF"
            # "Time\nCOF\nFF\nTemp"
            n2068 = case shown="True" w2320 {
              tunnel: [w2467 w2468] -> w2321
              frame False {
                n2069 = local read "string1"() -> (w2467:string)
              }
              frame True {
                n2070 = local read "String Indicator 4"() -> (w2468:string)
              }
            }
            n2071 = local read "string1 3"() -> (w2365:string)
            n2072 = String To Path(string=w2321) -> (path=w2452:path)
            n2073 = String To Path(string=w2365) -> (path=w2463:path)
            n2074 = local read "Numeric 12"() -> (w2449:i32)
            n2075 = local read "Numeric 8"() -> (w2451:i32)
            n2076 = local read "string1 2"() -> (w2366:string)
            n2077 = local read "string1 4"() -> (w2364:string)
            n2078 = Open/Create/Replace File "Open File"(file path (use dialog)=w2452) -> (refnum out=w2466:refnum<file>, error out=w2465:errorcluster)  [unwired: 5 in, 1 out]
            n2079 = Open/Create/Replace File "Open File"(file path (use dialog)=w2463) -> (refnum out=w2459:refnum<file>, error out=w2460:errorcluster)  [unwired: 5 in, 1 out]
            n2080 = for {
              N: w2451 -> [_]
              tunnel: w2466 -> [w2614]
              tunnel: w2465 -> [w2613]
              tunnel: [w2603] -> w2378 mode=indexing
              tunnel: [w2601] -> w2435 mode=indexing
              tunnel: [w2602] -> w2430 mode=indexing
              tunnel: w2447 -> [_]
              tunnel: [w2595] -> w2432 mode=indexing
              tunnel: [w2591] -> w2401 mode=indexing
              tunnel: [w2587] -> w2376 mode=indexing
              tunnel: [w2583] -> w2357 mode=indexing
              tunnel: [w2578] -> w2317 mode=indexing
              (unwired) TRUE ("line mode (F)")
              # "freq"
              # "Stroke"
              # "Time"
              # "CoF"
              # "Humidity"
              # "Temp"
              # "Air Temp"
              # "ECR"
              n2081 = Read from Text File "Read File"(file (use dialog)=w2614, error in=w2613) -> (text=w2579:string)  [unwired: 2 in, 3 out]
              n2082 = local write "String 6"(w2579) -> ()
              n2083 = String Subset(string=w2579, offset (0)=0, length (rest)=14 ("length (rest)")) -> (substring=w2607:string)
              n2084 = String Subset(string=w2579, offset (0)=35, length (rest)=9 ("length (rest)")) -> (substring=w2604:string)
              n2085 = String Subset(string=w2579, offset (0)=15, length (rest)=9 ("length (rest)")) -> (substring=w2610:string)
              n2086 = Fract/Exp String To Number(string=w2607) -> (number=w2603:dbl)  [unwired: 3 in, 1 out]
              n2087 = Fract/Exp String To Number(string=w2604) -> (number=w2602:dbl)  [unwired: 3 in, 1 out]
              n2088 = Fract/Exp String To Number(string=w2610) -> (number=w2601:dbl)  [unwired: 3 in, 1 out]
              n2089 = String Subset(string=w2579, offset (0)=85, length (rest)=9 ("length (rest)")) -> (substring=w2580:string)
              n2090 = String Subset(string=w2579, offset (0)=25, length (rest)=9 ("length (rest)")) -> (substring=w2586:string)
              n2091 = String Subset(string=w2579, offset (0)=55, length (rest)=9 ("length (rest)")) -> (substring=w2588:string)
              n2092 = String Subset(string=w2579, offset (0)=45, length (rest)=9 ("length (rest)")) -> (substring=w2594:string)
              n2093 = String Subset(string=w2579, offset (0)=65, length (rest)=9 ("length (rest)")) -> (substring=w2600:string)
              n2094 = Fract/Exp String To Number(string=w2586) -> (number=w2583:dbl)  [unwired: 3 in, 1 out]
              n2095 = Fract/Exp String To Number(string=w2580) -> (number=w2578:dbl)  [unwired: 3 in, 1 out]
              n2096 = Fract/Exp String To Number(string=w2588) -> (number=w2587:dbl)  [unwired: 3 in, 1 out]
              n2097 = Fract/Exp String To Number(string=w2594) -> (number=w2591:dbl)  [unwired: 3 in, 1 out]
              n2098 = Fract/Exp String To Number(string=w2600) -> (number=w2597:dbl)  [unwired: 3 in, 1 out]
              n2099 = Add(x=w2597, y=0.0) -> (x+y=w2595:dbl)
            }
            n2100 = for {
              N: w2449 -> [_]
              tunnel: w2460 -> [w2540]
              tunnel: w2459 -> [w2539]
              tunnel: [w2529] -> w2418 mode=indexing
              tunnel: [w2527] -> w2416 mode=indexing
              tunnel: [w2528] -> w2412 mode=indexing
              tunnel: w2447 -> [_]
              tunnel: [w2521] -> w2414 mode=indexing
              tunnel: [w2517] -> w2396 mode=indexing
              tunnel: [w2513] -> w2372 mode=indexing
              tunnel: [w2510] -> w2353 mode=indexing
              tunnel: [w2506] -> w2312 mode=indexing
              (unwired) 9 ("length (rest)")
              (unwired) 9 ("length (rest)")
              (unwired) TRUE ("line mode (F)")
              n2101 = Read from Text File "Read File"(file (use dialog)=w2539, error in=w2540) -> (text=w2507:string)  [unwired: 2 in, 3 out]
              n2102 = local write "String 8"(w2507) -> ()
              n2103 = String Subset(string=w2507, offset (0)=85) -> (substring=w2509:string)  [unwired: 1 in]
              n2104 = String Subset(string=w2507, offset (0)=35, length (rest)=9 ("length (rest)")) -> (substring=w2530:string)
              n2105 = String Subset(string=w2507, offset (0)=55, length (rest)=9 ("length (rest)")) -> (substring=w2515:string)
              n2106 = String Subset(string=w2507, offset (0)=25) -> (substring=w2511:string)  [unwired: 1 in]
              n2107 = String Subset(string=w2507, offset (0)=15, length (rest)=9 ("length (rest)")) -> (substring=w2536:string)
              n2108 = String Subset(string=w2507, offset (0)=0, length (rest)=14 ("length (rest)")) -> (substring=w2533:string)
              n2109 = String Subset(string=w2507, offset (0)=45, length (rest)=9 ("length (rest)")) -> (substring=w2520:string)
              n2110 = String Subset(string=w2507, offset (0)=65, length (rest)=9 ("length (rest)")) -> (substring=w2526:string)
              n2111 = Fract/Exp String To Number(string=w2509) -> (number=w2506:dbl)  [unwired: 3 in, 1 out]
              n2112 = Fract/Exp String To Number(string=w2530) -> (number=w2528:dbl)  [unwired: 3 in, 1 out]
              n2113 = Fract/Exp String To Number(string=w2515) -> (number=w2513:dbl)  [unwired: 3 in, 1 out]
              n2114 = Fract/Exp String To Number(string=w2511) -> (number=w2510:dbl)  [unwired: 3 in, 1 out]
              n2115 = Fract/Exp String To Number(string=w2536) -> (number=w2527:dbl)  [unwired: 3 in, 1 out]
              n2116 = Fract/Exp String To Number(string=w2533) -> (number=w2529:dbl)  [unwired: 3 in, 1 out]
              n2117 = Fract/Exp String To Number(string=w2520) -> (number=w2517:dbl)  [unwired: 3 in, 1 out]
